vi "Test Command.vi"() -> ()   [LabVIEW 2015]
uses:
  <vilib>/Instr/_visa.llb/VISA Configure Serial Port (Instr).vi
panel:
  out "read buffer":string
  out "length":string
  in  "Get Data":bool
  out "concatenated string 2":string
  out "hex integer string":string
  out "Array":string[](array[string])
  out "width (-)":u16 format="%.0b"
  out "x .and. y?":u16 format="%.0x"
  out "concatenated string":string
  in  "Command Channel":i32
  in  "Command ID":i32
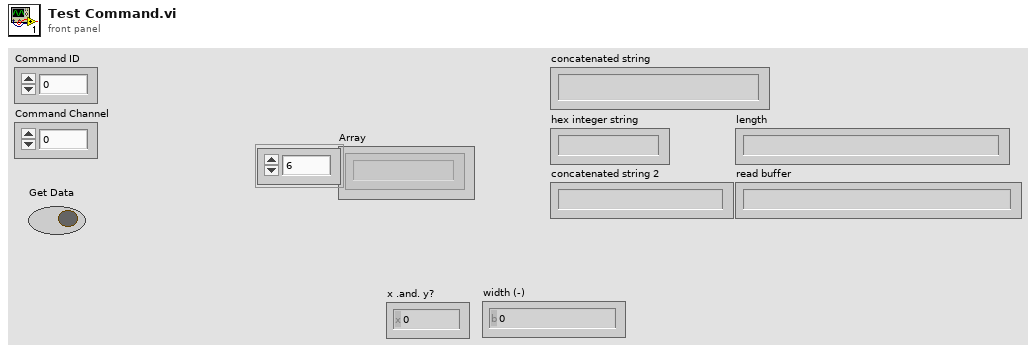
[diagram p1: front panel]
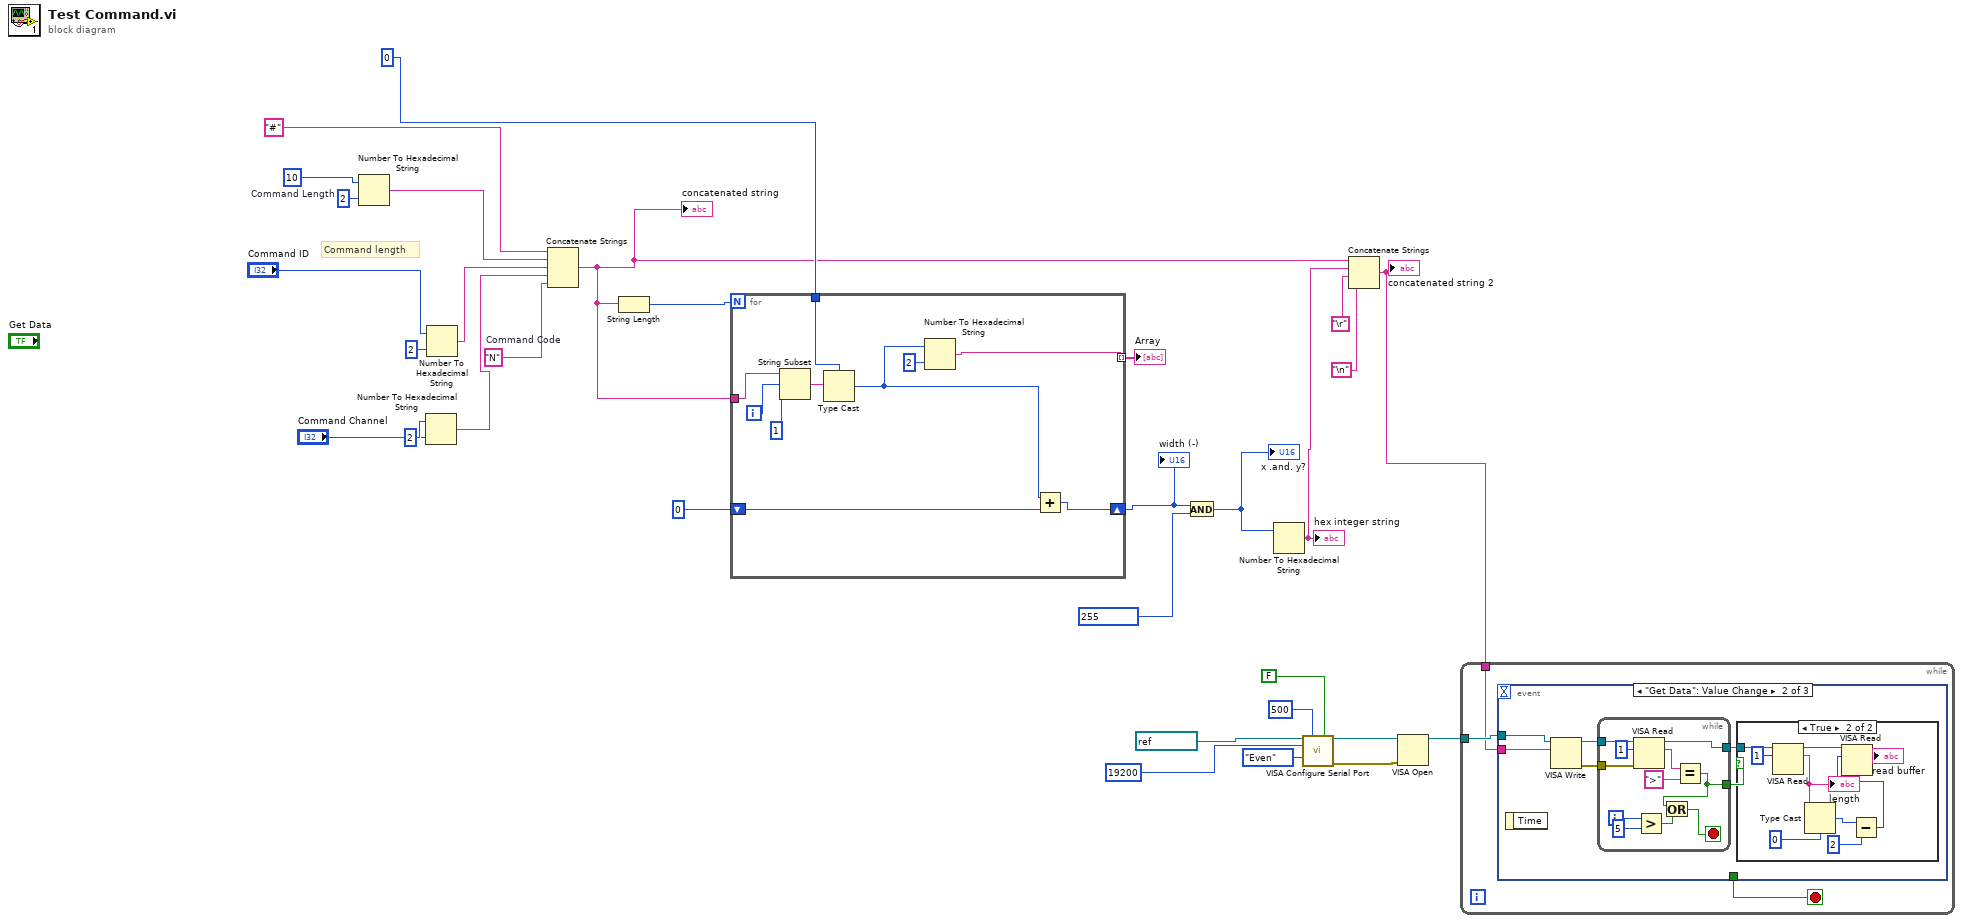
[diagram p0: block diagram]
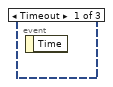
[diagram p2: hidden frame]
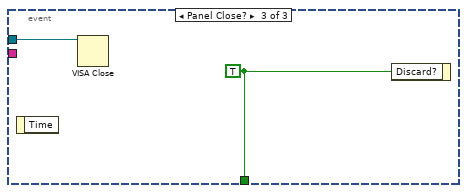
[diagram p4: hidden frame]
diagram:
  w26 = "N"  # Command Code
  w31 = 10  # Command Length
  # "Command length"
  n1 = Number To Hexadecimal String(1:i16 2 ("width (-)"), 2:w31) -> (0:w27:string)
  n2 = Number To Hexadecimal String(1:i16 2 ("width (-)"), 2:"Command Channel") -> (0:w22:string)
  n3 = Number To Hexadecimal String(1:i16 2 ("width (-)"), 2:"Command ID") -> (0:w23:string)
  n4 = Concatenate Strings("#", w27, w23, w22, w26) -> (w13:string)
  "concatenated string" <- w13
  n5 = String Length(string=w13) -> (length=w20:i32)
  n6 = for {
    N: w20 -> [_]
    tunnel: w13 -> [w41]
    tunnel: u8 0 ("output 2") -> [w38]
    shift-right: [w34] -> w17
    shift-left: u16 0 ("width (-)") -> [w35]
    tunnel: [w33] -> w15 mode=indexing
    i -> [w40]
    n7 = String Subset(string=w41, offset (0)=w40, length (rest)=1 ("length (rest)")) -> (substring=w37:string)
    n8 = Type Cast(type=w38, x=w37) -> (*(type *) &x=w32:u8)
    n9 = Number To Hexadecimal String(1:i16 2 ("width (-)"), 2:w32) -> (0:w33:string)
    n10 = Add(x=w32, y=w35) -> (x+y=w34:u16)
  }
  "width (-)" <- w17
  "Array" <- w15
  n11 = And(x=w17, y=u16 255) -> (x .and. y?=w14:u16)
  "x .and. y?" <- w14
  n12 = Number To Hexadecimal String(2:w14) -> (0:w12:string)  [unwired: 1 in]
  "hex integer string" <- w12
  n13 = call-poly "VISA Configure Serial Port"("VISA resource name"=refnum<visa-resource-name> "COM5", "timeout (10sec)"=u32 500, "Enable Termination\nChar (T)"=FALSE ("Enable Termination\nChar (T)"), "baud rate (9600)"=u32 19200, "parity (0:none)"=enum16{"None", "Odd", "Even", "Mark", "Space"}."Even") -> ("VISA resource name out"=w6:refnum<visa-resource-name>, "error out"=w5:errorcluster)  [unwired: 9 in]
  n14 = Concatenate Strings(w13, w12, "\r", "\n") -> (w1:string)
  "concatenated string 2" <- w1
  n15 = VISA Open(error in (no error)=w5, VISA resource name=w6) -> (VISA resource name=w4:refnum<visa-resource-name>)  [unwired: 3 in, 1 out]
  n16 = while {
    tunnel: w4 -> [w44]
    tunnel: w1 -> [w42]
    stop <- w43 stop-if-true
    n17 = event shown="[1] \"Get Data\": Value Change" {
      selector: _ -> [_ _ _]
      dyn-events: _ -> [_ _ _]
      timeout: _ -> [_ _ _]
      tunnel: w44 -> [_ w50 w71]
      tunnel: [_ _ w72] -> w43
      tunnel: w42 -> [_ w49 _]
      event Timeout {
        n18 = event-data() -> ()  [unwired: 1 in, 1 out]
      }
      event "Get Data": Value Change {
        n19 = event-data() -> ()  [unwired: 1 in, 1 out]
        n20 = VISA Write(VISA resource name=w50, write buffer=w49) -> (VISA resource name out=w48:refnum<visa-resource-name>, error out=w47:errorcluster)  [unwired: 1 in, 1 out]
        n21 = while {
          tunnel: w48 -> [w70]
          tunnel: w47 -> [w63]
          tunnel: [w62] -> w46
          tunnel: [w60] -> w45
          i -> [w68]
          stop <- w64 stop-if-true
          n22 = VISA Read(VISA resource name=w70, byte count=u32 1, error in (no error)=w63) -> (VISA resource name out=w62:refnum<visa-resource-name>, read buffer=w66:string)  [unwired: 2 out]
          n23 = Greater?(x=w68, y=5) -> (0:w61:bool)
          n24 = Equal?(x=w66, y=">") -> (x = y?=w60:bool)
          n25 = Or(x=w60, y=w61) -> (x .or. y?=w64:bool)
        }
        n26 = case shown="True" w45 {
          tunnel: w46 -> [_ w59]
          frame False {
          }
          frame True {
            n27 = VISA Read(VISA resource name=w59, byte count=u32 1) -> (VISA resource name out=w57:refnum<visa-resource-name>, read buffer=w52:string)  [unwired: 1 in, 2 out]
            "length" <- w52
            n28 = Type Cast(type=u8 0 ("byte count"), x=w52) -> (*(type *) &x=w55:u8)
            n29 = Subtract(x=w55, y=u32 2) -> (x-y=w53:u32)
            n30 = VISA Read(VISA resource name=w57, byte count=w53) -> (read buffer=→"read buffer":string)  [unwired: 1 in, 3 out]
          }
        }
      }
      event Panel Close? {
        w72 = TRUE ("Discard?")
        n31 = event-data() -> ()  [unwired: 1 in, 1 out]
        n32 = VISA Close(VISA resource name=w71) -> ()  [unwired: 1 in, 1 out]
        n33 = event-data("Discard?"=w72) -> ()  [unwired: 1 in, 1 out]
      }
    }
  }
